vi "Get ELVIS III PIDs.vi"() -> (3 "ELVIS III PIDs":u32[](array[numeric]) format="%.0x")   [LabVIEW 2021]
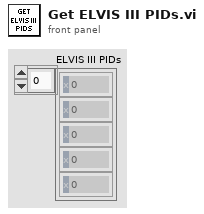
[diagram p1: front panel]
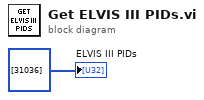
[diagram p0: block diagram]
diagram:
  "ELVIS III PIDs" <- u32[] [31036]
